vi "File Transfer To a Storage Device.vi"(7 "File Name ()":string, 8 "error in (no error)":errorcluster, 9 "Data Block Array (0)":i32, 10 "Data Block Size (0)":i32, 11 "VISA resource name":refnum<visa-resource-name>) -> (0 "error out":errorcluster, 3 "VISA resource name out":refnum<visa-resource-name>)   [LabVIEW 2018, in "Agilent ENA Series.lvlib"]
doc: "Writes data to a file on the built-in storage device of the E5070B/E5071B/E5071C.\n\nBy reading out data with this function and writing it to a file on the external controller, file transfer from the E5070B/E5071B/E5071C to the external controller can be realized. On the other hand, by reading out data from the external controller and writing it to a file on the E5070B/E5071B/E5071C with this function, file transfer from the external controller to the E5070B/E5071B/E5071C can be realized.\n\nSpecify the file name with the extension. If you want to specify a file on the floppy disk drive, you need to add \"A:\" at the beginning of the file name. When you use directory names and file name, separate them with \"/\" (slash) or \"\\\" (backslash)."
uses:
  Agilent ENA Series.lvlib
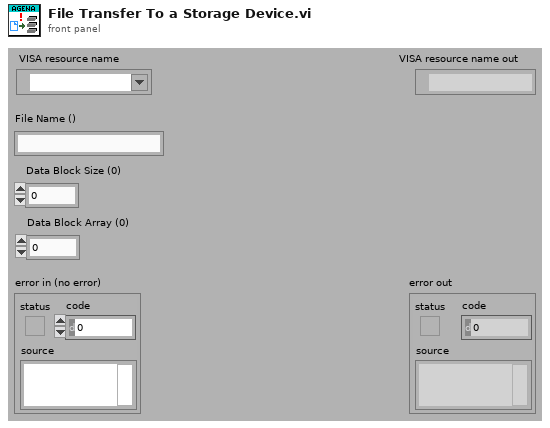
[diagram p1: front panel]
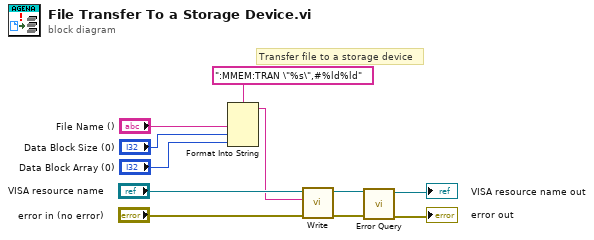
[diagram p0: block diagram]
diagram:
  # "Transfer file to a storage device"
  n1 = Format Into String(format string=":MMEM:TRAN \"%s\",#%ld%ld", "File Name ()", "Data Block Size (0)", "Data Block Array (0)") -> (resulting string=w7:string)  [unwired: 2 in, 1 out]
  n2 = call "Write.vi"("error in (no error)"="error in (no error)", "String ()"=w7, "VISA resource name"="VISA resource name") -> ("error out"=w3:errorcluster, "VISA resource name out"=w4:refnum<visa-resource-name>)  [unwired: 6 in, 1 out]
  n3 = call "Error Query.vi"("error in (no error)"=w3, "VISA resource name"=w4) -> ("error out"=→"error out":errorcluster, "VISA resource name out"=→"VISA resource name out":refnum<visa-resource-name>)  [unwired: 6 in, 2 out]
